vi "T1 Parametric Testing Retrieval.vi"(4 "error in (no error)":errorcluster, 6 "table name":string="Test_Results", 7 "connection reference":T1) -> (0 "error out":errorcluster, 3 "connection reference out":T1)   [LabVIEW 2013]
doc: "The T1 Parametric testing application performs parametric testing of T1 signals. The T1 signal is a 1.544 Mb/s pulsed digital signal formed by multiplexing 24 voice channels. Each channel is sampled at 8000 samples/sec. Each sample is then converted to 8 bits using Pulse Coded Multiplexing. The 24 channels are then time-division multiplexed. Each frame, which corresponds to one sampling period, contains 192 bits ( 8 times 24) plus one bit for frame synchronization. Since frames occur at 8000 times per second, the bit rate is 1.544 Mb/s\n\nThis application performs the following parametric tests on T1 signals:\n\n1. Mask Test: Compares T1 signals with standard masks. The type of masks that are supported are ITU G.703 mask, EIA/TIA 547 and ANSI T1.102. The graph shows the mask in grey, the actual signal in green and failures as red squares. A boolean indicates whether the signal passed or failed the mask test and the indicator Number of Hits shows the number of times the signal did not pass the mask test.\n\n2. Measure T1 signal amplitude : Measures the amplitude of the T1 signal. The peak amplitude is displayed in the indicator Measured Amplitude.\n\n3. Measure T1 signal frequency : Measures the frequency of the T1 signal. The signal frequency in MHz is displayed in the indicator Measured Frequency."
uses:
  Connection.llb/Conn ObjectReference.ctl
  Connection.llb/Conn Execute.vi
  Recordset.llb/Rec Fetch Recordset Data (R).vi
  Recordset.llb/Rec Destroy - Connection.vi
  Recordset.llb/Rec Save Recordset To File (R).vi
  _DB Variant To Data/Database Variant To Data.xnode
  NI_Database_API_64.lvlib
panel:
  in  "Sort By":u16(ring) items=["Operator", "Date/Time", "UUT Serial #", "Pass/Fail"]
  in  "File Name":string="C:\\test data.xml"
  in  "Order":bool=TRUE
  out "Database Data":i32(listbox)=-1
  in  "quit":bool
  in  "Retrieve Only Failures":bool
  in  "Retrieve All Data":bool
  in  "Sort Data":bool
  in  "Export All Data to XML":bool
  # "Telecommunications Parametric Testing Data Retrieval"
  # "Ascend."
  # "Descend."
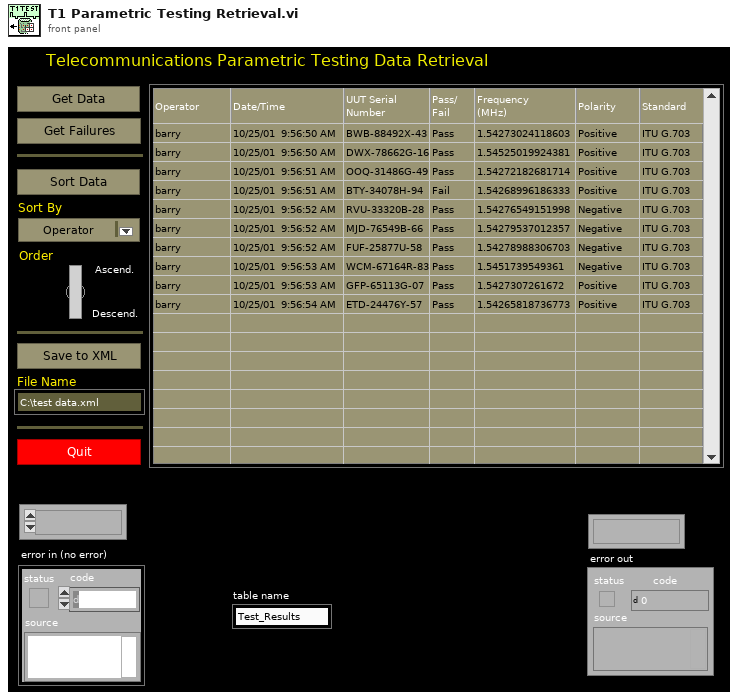
[diagram p1: front panel]
types:
  T1 = typedef "NI_Database_API_64.lvlib/Conn ObjectReference.ctl" = refnum<k1>
  T2 = typedef "NI_Database_API_64.lvlib/Rec ObjectReference.ctl" = refnum<k1>
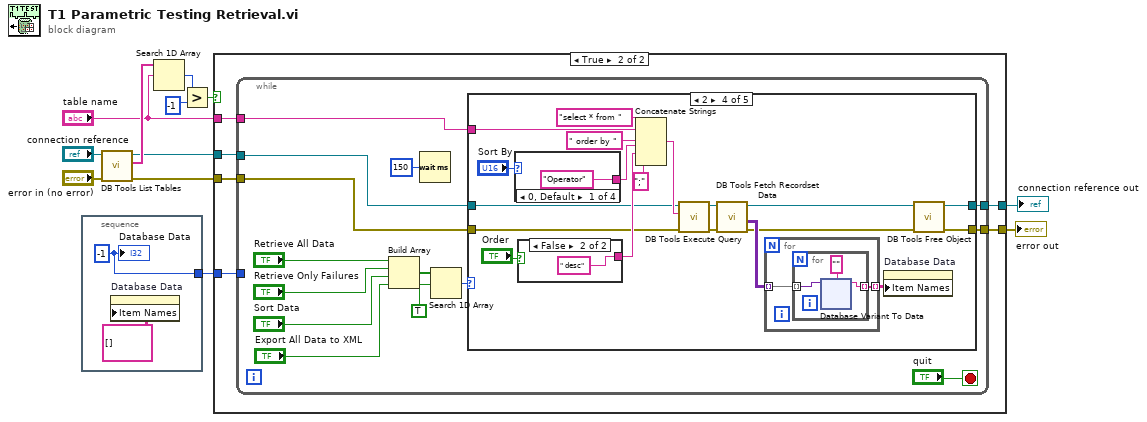
[diagram p0: block diagram]
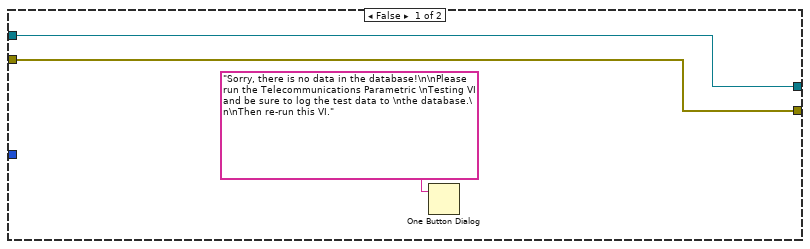
[diagram p2: hidden frame]
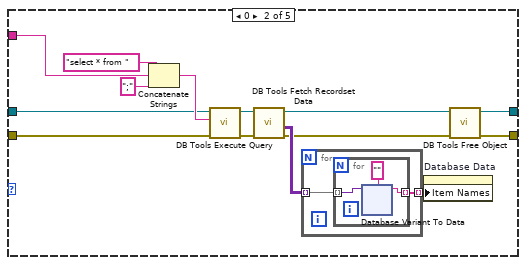
[diagram p4: hidden frame]
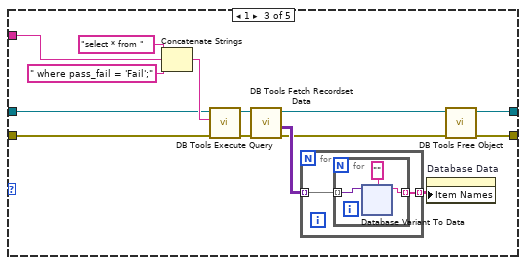
[diagram p5: hidden frame]
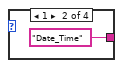
[diagram p6: hidden frame]
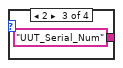
[diagram p7: hidden frame]
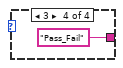
[diagram p8: hidden frame]
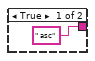
[diagram p9: hidden frame]
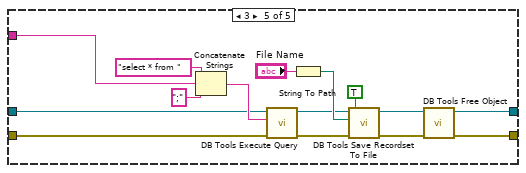
[diagram p10: hidden frame]
diagram:
  n1 = stacked-sequence {
    tunnel: [w14] -> w12
    frame #0 {
      w14 = -1 ("Database Data")
      n2 = property on="Database Data" class="MCListbox (strict)"("Item Names"=string[][] []) -> ()  [unwired: 2 in, 2 out]
      "Database Data" <- w14
    }
  }
  n3 = call "DB Tools List Tables.vi"("error in (no error)"="error in (no error)", "connection reference"="connection reference") -> ("error out"=w8:errorcluster, "tables"=w6:string[], "connection reference out"=w3:T1)  [unwired: 3 in]
  n4 = Search 1D Array(1D array=w6, element="table name") -> (index of element=w9:i32)  [unwired: 1 in]
  n5 = Greater?(x=w9, y=-1) -> (0:w1:bool)
  n6 = case shown="True" w1 {
    tunnel: w12 -> [_ w23]
    tunnel: [w16 w22] -> w10
    tunnel: [w15 w21] -> w11
    tunnel: "table name" -> [_ w20]
    tunnel: w3 -> [w16 w19]
    tunnel: w8 -> [w15 w18]
    frame False {
      n7 = One Button Dialog(message="Sorry, there is no data in the database!\n\nPlease run the Telecommunications Parametric \nTesting VI and be sure to log the test data to \nthe database.\n\nThen re-run this VI.") -> ()  [unwired: 1 in, 1 out]
    }
    frame True {
      n8 = while {
        tunnel: w20 -> [w25]
        tunnel: w18 -> [w26]
        tunnel: w19 -> [w27]
        tunnel: [w28] -> w21
        tunnel: [w29] -> w22
        tunnel: w23 -> [_]
        stop <- "quit" stop-if-true
        n9 = Build Array("Retrieve All Data", "Retrieve Only Failures", "Sort Data", "Export All Data to XML") -> (w32:bool[])
        n10 = Wait (ms)(milliseconds to wait=u32 150) -> ()  [unwired: 1 out]
        n11 = Search 1D Array(1D array=w32, element=TRUE) -> (index of element=w30:i32)  [unwired: 1 in]
        n12 = case shown="2" w30 {
          tunnel: w25 -> [_ w46 w97 w148 w210]
          tunnel: w27 -> [w39 w45 w96 w147 w209]
          tunnel: [w39 w41 w92 w143 w205] -> w29
          tunnel: [w38 w40 w91 w142 w204] -> w28
          tunnel: w26 -> [w38 w44 w95 w146 w208]
          frame -1, Default {
          }
          frame 0 {
            n13 = Concatenate Strings("select * from " ("SQL query"), w46, ";" ("Substring")) -> (w53:string)
            n14 = call-poly "DB Tools Execute Query.vi"("error in (no error)"=w44, "SQL query"=w53, "connection reference"=w45) -> ("error out"=w49:errorcluster, "recordset reference"=w50:T2)  [unwired: 5 in]
            n15 = call-poly "DB Tools Fetch Recordset Data.vi"("error in (no error)"=w49, "recordset reference"=w50) -> ("error out"=w42:errorcluster, "recordset data"=w48:variant[][], "recordset reference out"=w43:T2)  [unwired: 3 in]
            n16 = for {
              tunnel: w48 -> [w55] mode=indexing
              tunnel: [w54] -> w47 mode=indexing
              n17 = for {
                tunnel: w55 -> [w58] mode=indexing
                tunnel: [w56] -> w54 mode=indexing
                n18 = xnode "Database Variant To Data"("database variant"=w58, "type"="") -> ("data"=w56:string)  [unwired: 1 in, 1 out]
              }
            }
            n19 = property on="Database Data" class="MCListbox (strict)"("Item Names"=w47) -> ()  [unwired: 2 in, 2 out]
            n20 = call-poly "DB Tools Free Object.vi"("error in (no error)"=w42, "recordset reference"=w43) -> ("error out"=w40:errorcluster, "connection reference"=w41:T1)  [unwired: 8 in]
          }
          frame 1 {
            n21 = Concatenate Strings("select * from " ("SQL query"), w97, " where pass_fail = 'Fail';" ("Substring")) -> (w104:string)
            n22 = call-poly "DB Tools Execute Query.vi"("error in (no error)"=w95, "SQL query"=w104, "connection reference"=w96) -> ("error out"=w100:errorcluster, "recordset reference"=w101:T2)  [unwired: 5 in]
            n23 = call-poly "DB Tools Fetch Recordset Data.vi"("error in (no error)"=w100, "recordset reference"=w101) -> ("error out"=w93:errorcluster, "recordset data"=w99:variant[][], "recordset reference out"=w94:T2)  [unwired: 3 in]
            n24 = for {
              tunnel: w99 -> [w106] mode=indexing
              tunnel: [w105] -> w98 mode=indexing
              n25 = for {
                tunnel: w106 -> [w109] mode=indexing
                tunnel: [w107] -> w105 mode=indexing
                n26 = xnode "Database Variant To Data"("database variant"=w109, "type"="") -> ("data"=w107:string)  [unwired: 1 in, 1 out]
              }
            }
            n27 = property on="Database Data" class="MCListbox (strict)"("Item Names"=w98) -> ()  [unwired: 2 in, 2 out]
            n28 = call-poly "DB Tools Free Object.vi"("error in (no error)"=w93, "recordset reference"=w94) -> ("error out"=w91:errorcluster, "connection reference"=w92:T1)  [unwired: 8 in]
          }
          frame 2 {
            n29 = case shown="0, Default" "Sort By" {
              tunnel: ["Operator" ("Substring") "Date_Time" ("Substring") "UUT_Serial_Num" ("Substring") "Pass_Fail" ("Substring")] -> w157
              frame 0, Default {
              }
              frame 1 {
              }
              frame 2 {
              }
              frame 3 {
              }
            }
            n30 = case shown="False" "Order" {
              tunnel: [" asc" ("Substring") " desc" ("Substring")] -> w160
              frame True {
              }
              frame False {
              }
            }
            n31 = Concatenate Strings("select * from " ("SQL query"), w148, " order by " ("Substring"), w157, w160, ";" ("Substring")) -> (w149:string)
            n32 = call-poly "DB Tools Execute Query.vi"("error in (no error)"=w146, "SQL query"=w149, "connection reference"=w147) -> ("error out"=w153:errorcluster, "recordset reference"=w152:T2)  [unwired: 5 in]
            n33 = call-poly "DB Tools Fetch Recordset Data.vi"("error in (no error)"=w153, "recordset reference"=w152) -> ("error out"=w144:errorcluster, "recordset data"=w154:variant[][], "recordset reference out"=w145:T2)  [unwired: 3 in]
            n34 = for {
              tunnel: w154 -> [w162] mode=indexing
              tunnel: [w161] -> w155 mode=indexing
              n35 = for {
                tunnel: w162 -> [w165] mode=indexing
                tunnel: [w163] -> w161 mode=indexing
                n36 = xnode "Database Variant To Data"("database variant"=w165, "type"="") -> ("data"=w163:string)  [unwired: 1 in, 1 out]
              }
            }
            n37 = property on="Database Data" class="MCListbox (strict)"("Item Names"=w155) -> ()  [unwired: 2 in, 2 out]
            n38 = call-poly "DB Tools Free Object.vi"("error in (no error)"=w144, "recordset reference"=w145) -> ("error out"=w142:errorcluster, "connection reference"=w143:T1)  [unwired: 8 in]
          }
          frame 3 {
            n39 = Concatenate Strings("select * from " ("SQL query"), w210, ";" ("Substring")) -> (w211:string)
            n40 = call-poly "DB Tools Execute Query.vi"("error in (no error)"=w208, "SQL query"=w211, "connection reference"=w209) -> ("error out"=w214:errorcluster, "recordset reference"=w215:T2)  [unwired: 5 in]
            n41 = String To Path(string="File Name") -> (path=w216:path)
            n42 = call-poly "DB Tools Save Recordset To File.vi"("overwrite? (F)"=TRUE ("overwrite? (f)"), "error in (no error)"=w214, "file name"=w216, "recordset reference"=w215) -> ("error out"=w206:errorcluster, "recordset reference out"=w207:T2)  [unwired: 4 in]
            n43 = call-poly "DB Tools Free Object.vi"("error in (no error)"=w206, "recordset reference"=w207) -> ("error out"=w204:errorcluster, "connection reference"=w205:T1)  [unwired: 8 in]
          }
        }
      }
    }
  }
  "connection reference out" <- w10
  "error out" <- w11
